vi "GetEventRef.vi"(10 "EQ_Name in":string, 11 "Data Value Reference in":refnum<data-value>) -> (2 "user event out":refnum<user-event>, 3 "Data Value Reference out":refnum<data-value>)   [LabVIEW 2014]
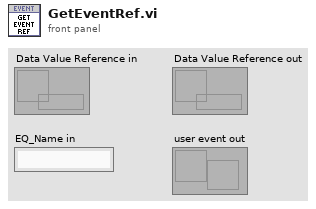
[diagram p1: front panel]
types:
  T1 = cluster{"CmdMsg":cluster{"msg":string, "data":variant}, "EQ_Name":string, "user event out":refnum<user-event>}[]
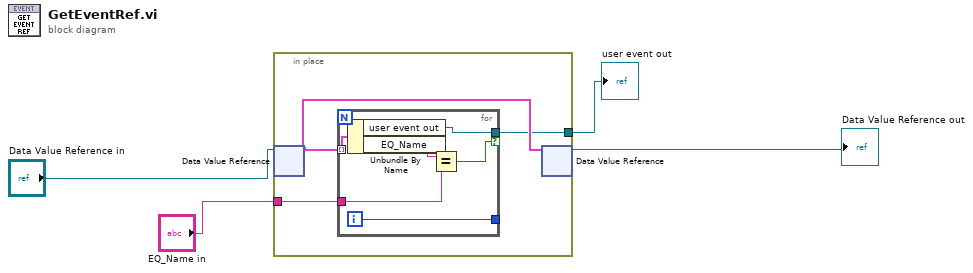
[diagram p0: block diagram]
diagram:
  n1 = in-place {
    in-place-border: [w6] -> w3
    in-place-border: "EQ_Name in" -> [w5]
    n2 = in-place-dvr #1("Data Value Reference in") -> (w7:T1)  [unwired: 1 out]
    n3 = for {
      tunnel: w7 -> [w13] mode=indexing
      tunnel: [w10] -> w6 if=w11
      tunnel: w5 -> [w9]
      tunnel: [w8] -> _
      i -> [w8]
      n4 = Unbundle By Name(w13) -> ("user event out"=w10:refnum<user-event>, "EQ_Name"=w12:string)
      n5 = Equal?(x=w12, y=w9) -> (x = y?=w11:bool)
    }
    n6 = in-place-dvr #1(w7) -> (→"Data Value Reference out":refnum<data-value>)  [unwired: 1 out]
  }
  "user event out" <- w3
